vi "Actor Core.vi"(8 "error in":errorcluster, 11 "Simple Chat in":refnum<class "Simple Chat.lvclass">) -> (0 "error out":errorcluster, 3 "Actor out":refnum<class "Actor.lvclass">)   [LabVIEW 2020, in "Simple Chat.lvlib" / "Simple Chat.lvclass"]
doc: "(<B>Filename</B>: Actor Framework.lvlib:Actor.lvclass:Actor Core.vi)\n\nReceives messages to the actor, reacts to them, and initiates any error handling that may shut the actor down.\n\nDescendant classes may override this VI to append parallel tasks for the actor to complete while it handles messages. Overrides use the Call Parent Class Method node."
uses:
  Simple Chat.lvclass
  C:/Program Files/National Instruments/LabVIEW 2020/vi.lib/ActorFramework/Actor/Actor.lvclass
  <vilib>/ActorFramework/Actor/Actor.lvclass
  <vilib>/ActorFramework/Actor/Actor.lvclass/Actor.ctl
  <vilib>/ActorFramework/Message Enqueuer/Message Enqueuer.lvclass/Message Enqueuer.ctl
  Simple Chat.lvclass/Simple Chat.ctl
  Message Reciever Interface/Message Reciever Interface.lvclass
  Simple Chat Messages/Recieve Message Msg/Recieve Message Msg.lvclass/Recieve Message Msg.ctl
  <vilib>/ActorFramework/Message Enqueuer/Init from Existing Queue.vi
  <vilib>/ActorFramework/Message Enqueuer/Enqueue.vi
  Simple Chat Messages/Recieve Message Msg/Recieve Message Msg.lvclass
  C:/Program Files/National Instruments/LabVIEW 2020/vi.lib/ActorFramework/Message/Message.lvclass
  <vilib>/ActorFramework/Stop Msg/Stop Msg.lvclass
  <vilib>/ActorFramework/Message Priority Queue/Priority Enqueue.vi
  <vilib>/ActorFramework/Message Enqueuer/Message Enqueuer.lvclass
  Actor Pub Sub Channels/Helpers/Unsubscribe Topic.vi
  Actor Pub Sub Channels/Helpers/Get Class Topic Enqueuer.vi
  Actor Pub Sub Channels/Actor Pub Sub Channels.lvlib
  E:/Labview/LV 2020/Libs/Actor Pub Sub/Source/Simple Chat/Simple Chat/Simple Chat.lvclass
  E:/Labview/LV 2020/Libs/Actor Pub Sub/Source/Actor Pub Sub Channels/PubSub Status Reciever Interface/PubSub Status Reciever Interface.lvclass
  E:/Labview/LV 2020/Libs/Actor Pub Sub/Source/Simple Chat/Message Reciever Interface/Message Reciever Interface.lvclass
panel:
  out "Messages":string
  in  "Message":string
  in  "OK Button":bool
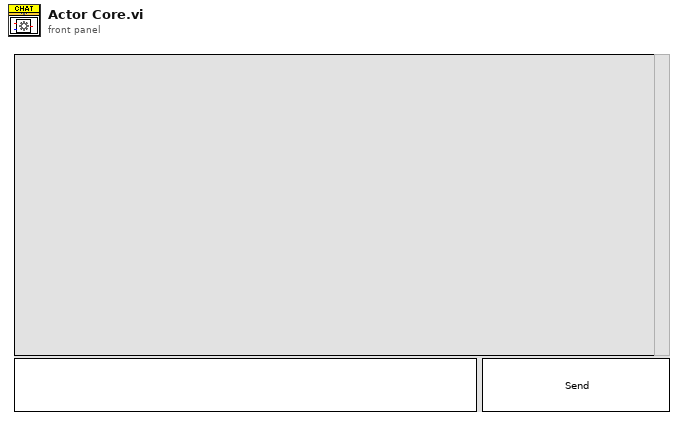
[diagram p1: front panel]
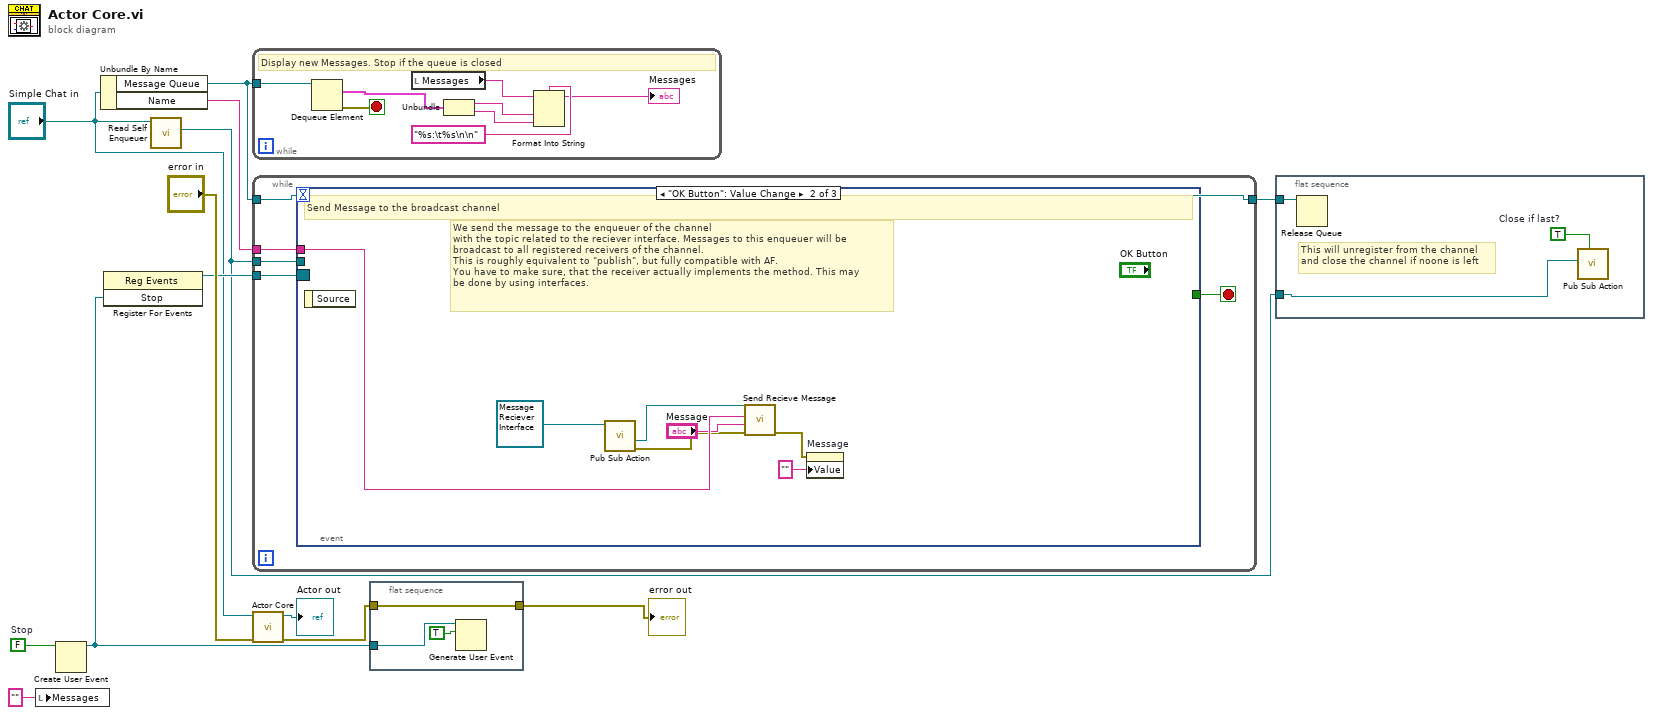
[diagram p0: block diagram]
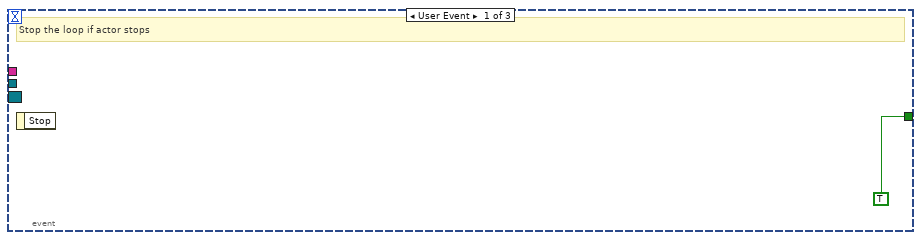
[diagram p2: hidden frame]
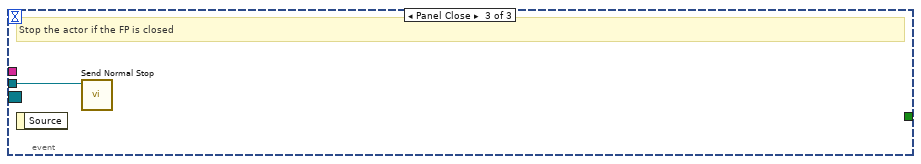
[diagram p3: hidden frame]
diagram:
  w3 = FALSE  # Stop
  n1 = local write "Messages"("" ("Messages")) -> ()
  n2 = Create User Event(user event datatype=w3) -> (user event=w2:refnum<user-event>)  [unwired: 1 in, 1 out]
  n3 = Unbundle By Name("Simple Chat in") -> ("Message Queue"=w9:refnum<queue>, "Name"=w10:string)
  n4 = register-events(w2) -> (reference out=w11:refnum<event-registration>)  [unwired: 2 in, 1 out]
  n5 = call <vilib>:"Read Self Enqueuer.vi"("Actor"="Simple Chat in") -> ("Self Enqueuer"=w5:refnum<class "Message Enqueuer.lvclass">)  [unwired: 10 in]
  n6 = while {
    tunnel: w9 -> [w21]
    stop <- w20 stop-if-true
    # "Display new Messages. Stop if the queue is closed"
    n7 = Dequeue Element(queue=w21) -> (element=w19:cluster{"Sender":string, "Message":string}, error out=w20:errorcluster)  [unwired: 2 in, 2 out]
    n8 = local read "Messages"() -> (w15:string)
    n9 = Unbundle(w19) -> ("Sender"=w18:string, "Message"=w17:string)
    n10 = Format Into String(format string="%s:\t%s\n\n", initial string=w15, w18, w17) -> (resulting string=→"Messages":string)  [unwired: 1 in, 1 out]
  }
  n11 = while {
    tunnel: w11 -> [w26]
    tunnel: w10 -> [w24]
    tunnel: w9 -> [w23]
    tunnel: [w23] -> w8
    tunnel: w5 -> [w22]
    stop <- w25 stop-if-true
    n12 = event shown="[1] \"OK Button\": Value Change" {
      selector: w26 -> [_ _ _]
      dyn-events: _ -> [_ _ _]
      timeout: _ -> [_ _ _]
      tunnel: [TRUE _ _] -> w25
      tunnel: w24 -> [_ w34 _]
      tunnel: w22 -> [_ _ w35]
      event User Event {
        # "Stop the loop if actor stops"
        n13 = event-data() -> ()  [unwired: 1 in, 1 out]
      }
      event "OK Button": Value Change {
        # "We send the message to the enqueuer of the channel \nwith the topic related to the reciever interface. Messages to this enqueuer will be\nbroadcast to all registered receivers of the channel. \nThis is roughly equivalent to \"publish\", but fully compatible with AF.\nYou have to make sure, that the receiver actually implements the method. This may\nbe done by using interfaces."
        # "Send Message to the broadcast channel"
        n14 = event-data() -> ()  [unwired: 1 in, 1 out]
        n15 = call-poly "Pub Sub Action.vi"("Topic"=refnum<class "Message Reciever Interface.lvclass"> refnum ("Simple Chat.lvlib:Message Reciever Interface.lvclass")) -> ("error out"=w28:errorcluster, "Topic Enqueuer"=w29:refnum<class "Message Enqueuer.lvclass">)  [unwired: 7 in, 2 out]
        n16 = call "Send Recieve Message.vi"("error in (no error)"=w28, "Message"="Message", "Sender"=w34, "Message Enqueuer"=w29) -> ("error out"=w32:errorcluster)  [unwired: 6 in, 1 out]
        n17 = property on="Message" class="Str"(error in=w32, "Value"="" ("Message")) -> ()  [unwired: 1 in, 2 out]
      }
      event Panel Close {
        # "Stop the actor if the FP is closed"
        n18 = event-data() -> ()  [unwired: 1 in, 1 out]
        n19 = call <vilib>:"Send Normal Stop.vi"("Message Enqueuer"=w35) -> ()  [unwired: 10 in, 1 out]
      }
    }
  }
  n20 = call-parent "Actor Core.vi"("error in"="error in", "Actor in"="Simple Chat in") -> ("error out"=w4:errorcluster, "Actor out"=→"Actor out":refnum<class "Actor.lvclass">)  [unwired: 8 in]
  n21 = flat-sequence {
    tunnel: w4 -> [w36]
    tunnel: w2 -> [w37]
    tunnel: [w36] -> w1
    frame #0 {
      n22 = Generate User Event(user event=w37, event data cluster=TRUE ("event data")) -> ()  [unwired: 2 in, 2 out]
    }
  }
  n23 = flat-sequence {
    tunnel: w8 -> [w41]
    tunnel: w5 -> [w40]
    frame #0 {
      w39 = TRUE  # Close if last?
      # "This will unregister from the channel\nand close the channel if noone is left"
      n24 = Release Queue(queue=w41) -> ()  [unwired: 2 in, 3 out]
      n25 = call-poly "Pub Sub Action.vi"("Close if last?"=w39, "Receivers Enqueuer"=w40) -> ()  [unwired: 9 in, 1 out]
    }
  }
  "error out" <- w1
